vi "MathUtil_Clamp.vi"(9 "High Limit":dbl, 10 "Low Limit":dbl, 11 "Value":dbl) -> (3 "Result":dbl)   [LabVIEW 2019, in "Trajectory_Library.lvlib"]
doc: "Returns value clamped between low and high boundaries.\n \nInputs:\n - value -- Value to clamp.\n - low limit -- The lower boundary to which to clamp value.\n - high limit -- The higher boundary to which to clamp value.\n\nOutputs:\n - Result -- The clamped value."
uses:
  Trajectory_Library.lvlib
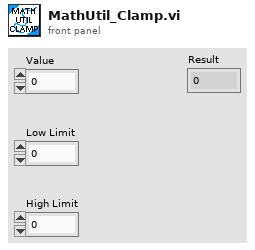
[diagram p1: front panel]
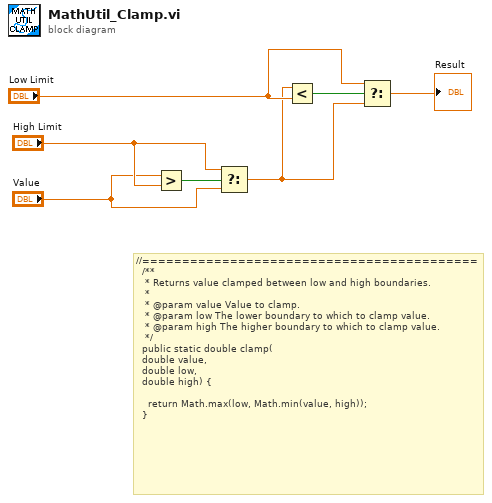
[diagram p0: block diagram]
diagram:
  # "//==========================================\n  /**\n   * Returns value clamped between low and high boundaries.\n   *\n   * @param value Value to clamp.\n   * @param low The lower boundary to which to clamp value.\n   * @param high The higher boundary to which to clamp value.\n   */\n  public static double clamp(\n\t\tdouble value, \n\t\tdouble low, \n\t\tdouble high) {\n\n    return Math.max(low, Math.min(value, high));\n  }"
  n1 = Greater?(x="Value", y="High Limit") -> (0:w6:bool)
  n2 = Select(t="High Limit", s=w6, f="Value") -> (s? t:f=w2:dbl)
  n3 = Less?(x=w2, y="Low Limit") -> (x < y?=w7:bool)
  n4 = Select(t="Low Limit", s=w7, f=w2) -> (s? t:f=→"Result":dbl)
